vi "configSampling.vi"(5 "Port":u16, 7 "address":string, 8 "error in (no error)":errorcluster, 10 "Sampling":T1={"Fs"=204789, "#s"=15753}, 11 "Instrument.Lockin in":refnum<class "Instrument.Lockin.lvclass">) -> (0 "error out":errorcluster, 3 "Instrument.Lockin out":refnum<class "Instrument.Lockin.lvclass">)   [LabVIEW 2016]
doc: "API to put lockin into remote mode.\n\nIf address=\"\", this API reads from localhost\nIf address is remote lockin, you need to add this computer to allowed whitelist on the lockin computer you are trying to access."
uses:
  Instrument.Lockin/Typedefs/Sampling.ctl
  Instrument.Lockin/Instrument.Lockin.lvclass
  Instrument.Lockin/Typedefs/Instrument.Lockin.Commands--Enum.ctl
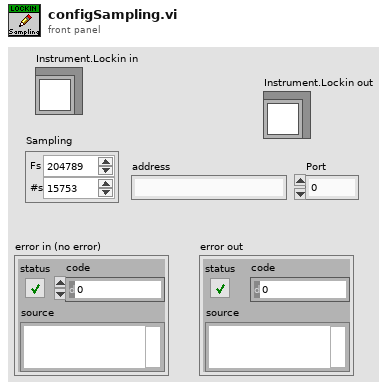
[diagram p1: front panel]
types:
  T1 = typedef "Instrument.Lockin.lvclass/Sampling.ctl" = cluster{"Fs":i32, "#s":i32}
  T2 = typedef "Instrument.Lockin.lvclass/Instrument.Lockin.Commands--Enum.ctl" = enum16{"configAO", "configAO_Amplitude", "configAO_DC", "configAO_Frequency", "configAO_Phase", "configAO_Function", "configAO_I+", "configREF", "configREF_Frequency", "configREF_Phase", "configREF_Filter", "configIVmode", "Reset", "configSampling", "Trigger", "getAO", "getAI", "getResults", "getTrigger", "getIVmode", "getSampling", "getAOconfig", "getREFconfig", "getREF_Filter", "configGain", "getGain", "configAutoSampling", "getAutoSampling"}
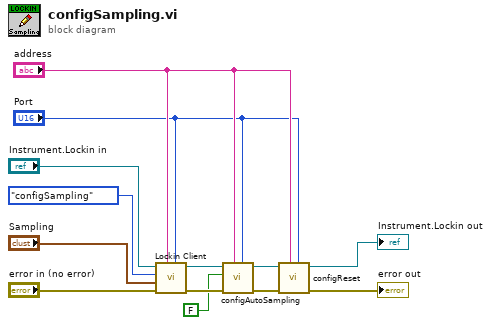
[diagram p0: block diagram]
diagram:
  n1 = call "Lockin Client.vi"("Port"="Port", "address"="address", "error in (no error)"="error in (no error)", "Data"="Sampling", "Command"=Instrument.Lockin.Commands--Enum."configSampling", "Instrument.Lockin in"="Instrument.Lockin in") -> ("error out"=w4:errorcluster, "Instrument.Lockin out"=w7:refnum<class "Instrument.Lockin.lvclass">)  [unwired: 3 in, 1 out]
  n2 = call "configAutoSampling.vi"("Port"="Port", "address"="address", "error in (no error)"=w4, "Auto Sampling"=FALSE, "Instrument.Lockin in"=w7) -> ("error out"=w3:errorcluster, "Instrument.Lockin out"=w2:refnum<class "Instrument.Lockin.lvclass">)  [unwired: 5 in]
  n3 = call "configReset.vi"("Port"="Port", "address"="address", "error in (no error)"=w3, "Instrument.Lockin in"=w2) -> ("error out"=→"error out":errorcluster, "Instrument.Lockin out"=→"Instrument.Lockin out":refnum<class "Instrument.Lockin.lvclass">)  [unwired: 6 in]
